vi "PeakDetect_FindShoulderIndexes.vi"(10 "2nd Deriv":dbl[](array[numeric]), 11 "Peaks Info":T1[](array[typedef])) -> (3 "Array":T1[](array[typedef]))   [LabVIEW 2015]
uses:
  Controls/PeakInfoPresenter.ctl
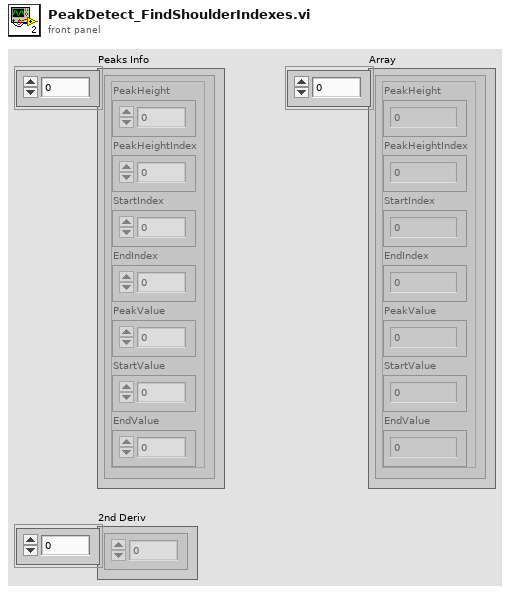
[diagram p1: front panel]
types:
  T1 = typedef "PeakInfoPresenter.ctl" = cluster{"PeakHeight":dbl, "PeakHeightIndex":dbl, "StartIndex":dbl, "EndIndex":dbl, "PeakValue":dbl, "StartValue":dbl, "EndValue":dbl}
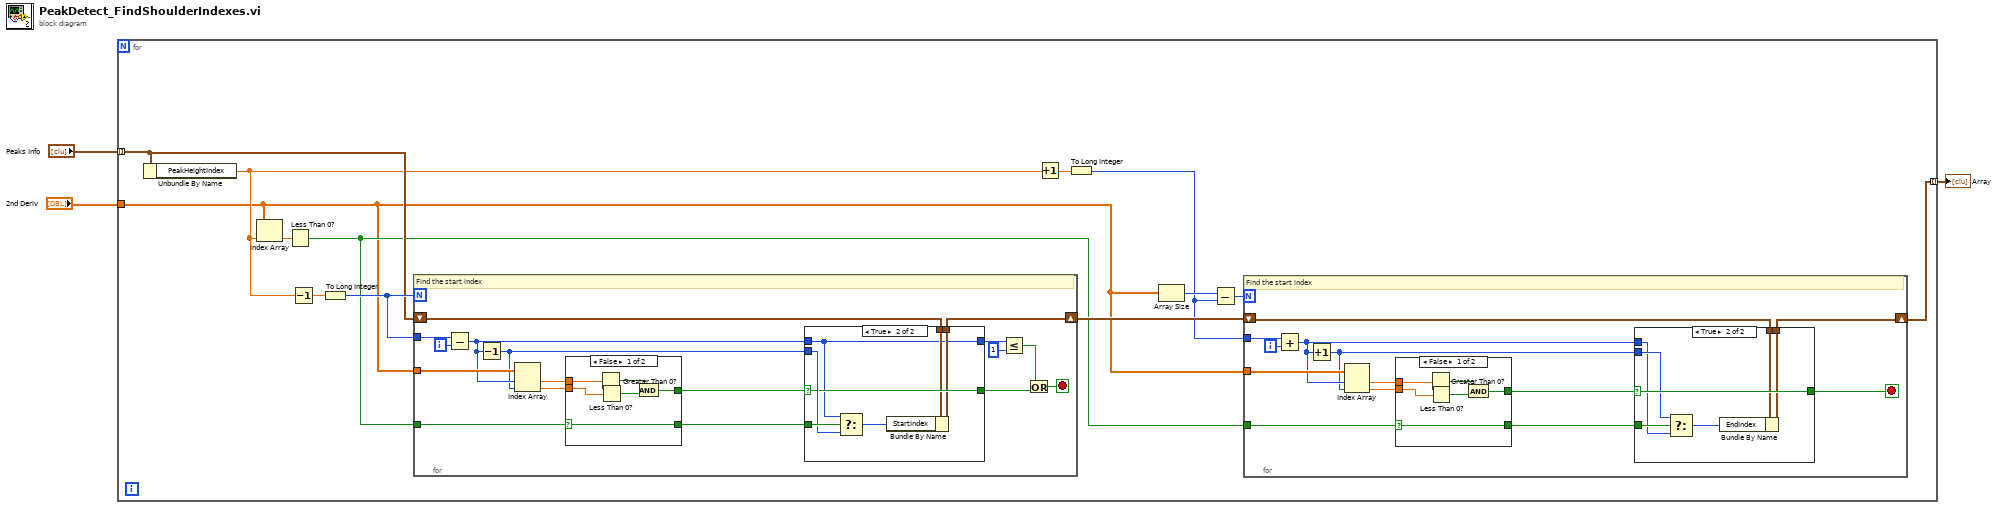
[diagram p0: block diagram]
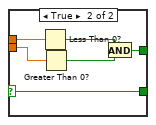
[diagram p3: hidden frame]
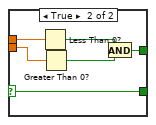
[diagram p5: hidden frame]
diagram:
  n1 = for {
    tunnel: "Peaks Info" -> [w13] mode=indexing
    tunnel: "2nd Deriv" -> [w7]
    tunnel: [w8] -> w1 mode=indexing
    n2 = Unbundle By Name(w13) -> ("PeakHeightIndex"=w9:dbl)
    n3 = Index Array(array=w7, index=w9) -> (element=w16:dbl)
    n4 = Less Than 0?(x=w16) -> (x < 0?=w11:bool)
    n5 = Decrement(x=w9) -> (x-1=w15:dbl)
    n6 = To Long Integer(number=w15) -> (32bit integer=w14:i32)
    n7 = for {
      N: w14 -> [_]
      tunnel: w7 -> [w65]
      tunnel: w14 -> [w67]
      tunnel: w11 -> [w64]
      shift-right: [w59] -> w12
      shift-left: w13 -> [w60]
      i -> [w66]
      stop <- w54 stop-if-true
      # "Find the start index"
      n8 = Subtract(x=w67, y=w66) -> (x-y=w57:i32)
      n9 = Decrement(x=w57) -> (x-1=w56:i32)
      n10 = Index Array(array=w65, index #1=w57, index #2=w56) -> (element #1=w63:dbl, element #2=w62:dbl)
      n11 = case shown="False" w64 {
        selector: w64 -> [w78 w84]
        tunnel: w63 -> [w81 w89]
        tunnel: w62 -> [w80 w88]
        tunnel: [w79 w85] -> w61
        tunnel: [w78 w84] -> w58
        frame False {
          n12 = Greater Than 0?(x=w81) -> (x > 0?=w83:bool)
          n13 = Less Than 0?(x=w80) -> (x < 0?=w82:bool)
          n14 = And(x=w83, y=w82) -> (x .and. y?=w79:bool)
        }
        frame True {
          n15 = Less Than 0?(x=w89) -> (x < 0?=w87:bool)
          n16 = Greater Than 0?(x=w88) -> (x > 0?=w86:bool)
          n17 = And(x=w87, y=w86) -> (x .and. y?=w85:bool)
        }
      }
      n18 = case shown="True" w61 {
        selector: w61 -> [w69 w75]
        tunnel: w60 -> [w70 w74]
        tunnel: [w70 w73] -> w59
        tunnel: w58 -> [_ w77]
        tunnel: w57 -> [w68 w71]
        tunnel: w56 -> [_ w76]
        tunnel: [w69 w75] -> w55
        tunnel: [w68 w71] -> w53
        frame False {
        }
        frame True {
          n19 = Select(t=w71, s=w77, f=w76) -> (s? t:f=w72:i32)
          n20 = Bundle By Name(cluster=w74, "StartIndex"=w72) -> (w73:T1)
        }
      }
      n21 = Less Or Equal?(x=w53, y=1) -> (x <= y?=w51:bool)
      n22 = Or(x=w51, y=w55) -> (x .or. y?=w54:bool)
    }
    n23 = Increment(x=w9) -> (x+1=w10:dbl)
    n24 = To Long Integer(number=w10) -> (32bit integer=w5:i32)
    n25 = Array Size(array=w7) -> (size(s)=w6:i32)
    n26 = Subtract(x=w6, y=w5) -> (x-y=w4:i32)
    n27 = for {
      N: w4 -> [_]
      tunnel: w7 -> [w27]
      tunnel: w5 -> [w29]
      tunnel: w11 -> [w26]
      shift-right: [w21] -> w8
      shift-left: w12 -> [w22]
      i -> [w28]
      stop <- w17 stop-if-true
      # "Find the start index"
      n28 = Add(x=w29, y=w28) -> (x+y=w19:i32)
      n29 = Increment(x=w19) -> (x+1=w18:i32)
      n30 = Index Array(array=w27, index #1=w19, index #2=w18) -> (element #1=w25:dbl, element #2=w24:dbl)
      n31 = case shown="False" w26 {
        selector: w26 -> [w39 w45]
        tunnel: w25 -> [w42 w50]
        tunnel: w24 -> [w41 w49]
        tunnel: [w40 w46] -> w23
        tunnel: [w39 w45] -> w20
        frame False {
          n32 = Greater Than 0?(x=w42) -> (x > 0?=w44:bool)
          n33 = Less Than 0?(x=w41) -> (x < 0?=w43:bool)
          n34 = And(x=w44, y=w43) -> (x .and. y?=w40:bool)
        }
        frame True {
          n35 = Less Than 0?(x=w50) -> (x < 0?=w48:bool)
          n36 = Greater Than 0?(x=w49) -> (x > 0?=w47:bool)
          n37 = And(x=w48, y=w47) -> (x .and. y?=w46:bool)
        }
      }
      n38 = case shown="True" w23 {
        selector: w23 -> [w30 w37]
        tunnel: w22 -> [w31 w36]
        tunnel: [w31 w35] -> w21
        tunnel: w20 -> [_ w38]
        tunnel: w19 -> [_ w32]
        tunnel: w18 -> [_ w33]
        tunnel: [w30 w37] -> w17
        frame False {
        }
        frame True {
          n39 = Select(t=w33, s=w38, f=w32) -> (s? t:f=w34:i32)
          n40 = Bundle By Name(cluster=w36, "EndIndex"=w34) -> (w35:T1)
        }
      }
    }
  }
  "Array" <- w1
